vi "Latest DAQmx timestamp.vi"() -> ()   [LabVIEW 2017]
panel:
  out "Latest DAQmx timestamp":timestamp
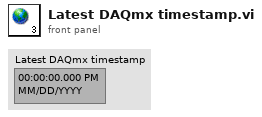
[diagram p1: front panel]
diagram:
